vi "Customizing the Menubar.vi"() -> ()   [LabVIEW 2014]
doc: "本VI演示如何通过编程添加和删除VI运行时菜单栏中的项。"
uses:
  <vilib>/Utility/miscctls.llb/LVMenuShortCut.ctl
panel:
  in  "删除首选项":bool
  in  "删除新建":bool
  out "已选菜单项标识符":string
  in  "停止":bool
  # "概述：演示使用菜单函数控制VI运行时菜单栏的内容。\n操作步骤：\n1. 运行VI。自定义“文件”和“编辑”菜单将出现在菜单栏中。\n2. 选择多个不同菜单项。选择将显示在已选菜单项标识符显示控件中。\n3. 单击两个删除按钮。注意“文件 > 新建”和“文件 > 首选项”菜单项已移除。\n4. 单击停止可停止VI。"
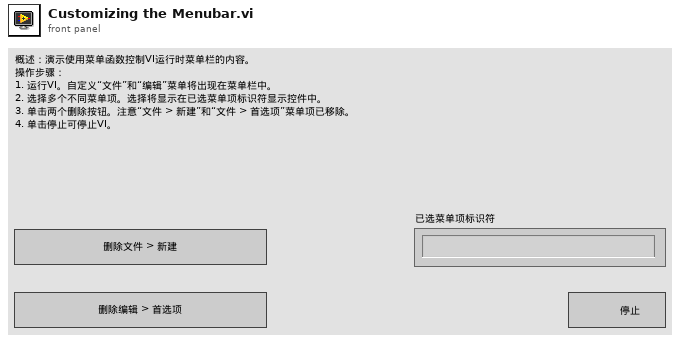
[diagram p1: front panel]
types:
  T1 = enum8{"Enabled", "Disabled", "Disabled and Grayed Out"}
  T2 = typedef "LVMenuShortCut.ctl" = cluster{"Include Shift Key?":bool, "Include Ctrl Key?":bool, "Shortcut Key":string}
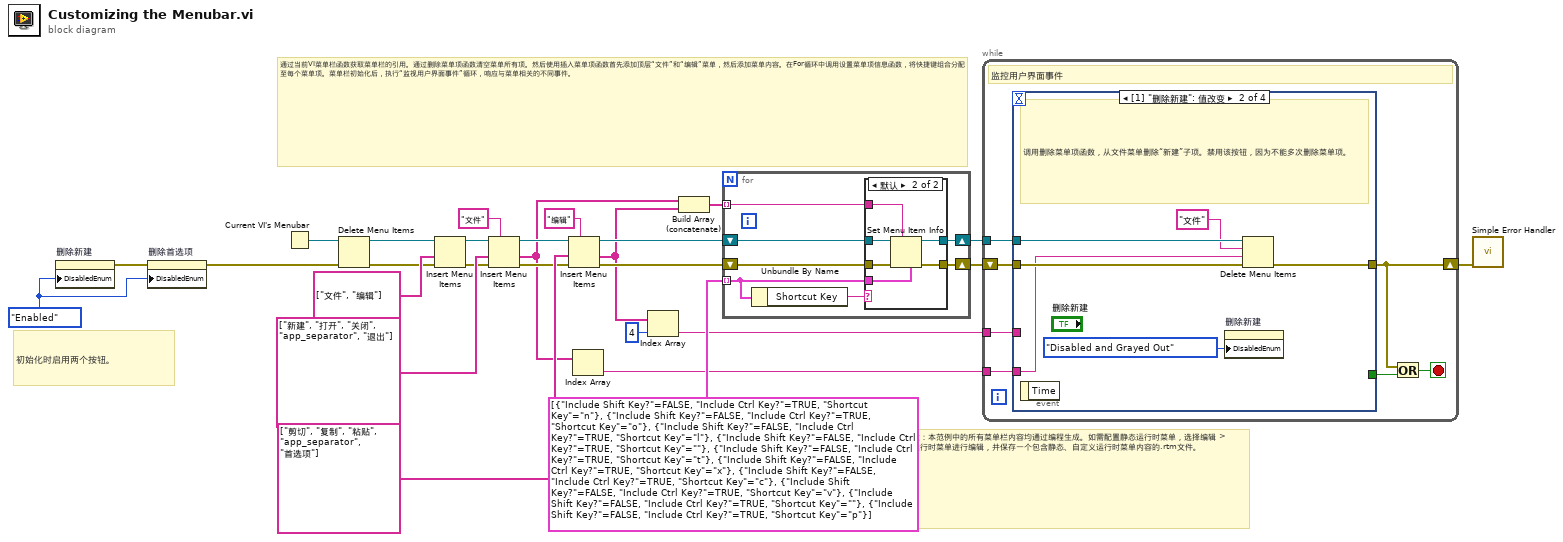
[diagram p0: block diagram]
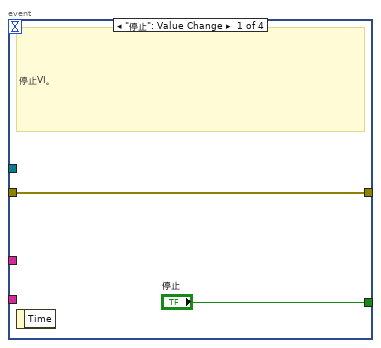
[diagram p2: hidden frame]
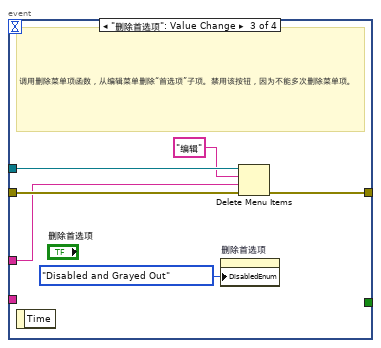
[diagram p3: hidden frame]
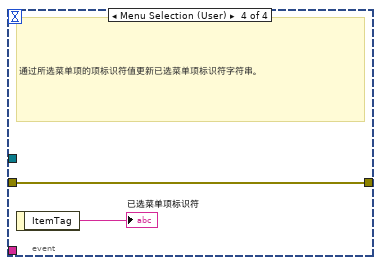
[diagram p4: hidden frame]
diagram:
  w1 = T1."Enabled" ("Disabled")
  # "注：本范例中的所有菜单栏内容均通过编程生成。如需配置静态运行时菜单，选择编辑 > 运行时菜单进行编辑，并保存一个包含静态、自定义运行时菜单内容的.rtm文件。"
  # "初始化时启用两个按钮。"
  # "通过当前VI菜单栏函数获取菜单栏的引用。通过删除菜单项函数清空菜单所有项。然后使用插入菜单项函数首先添加顶层“文件”和“编辑”菜单，然后添加菜单内容。在For循环中调用设置菜单项信息函数，将快捷键组合分配至每个菜单项。菜单栏初始化后，执行“监视用户界面事件”循环，响应与菜单相关的不同事件。"
  n1 = property on="删除新建" class="Bool"("DisabledEnum"=w1) -> (error out=w3:errorcluster)  [unwired: 2 in, 1 out]
  n2 = property on="删除首选项" class="Bool"(error in=w3, "DisabledEnum"=w1) -> (error out=w2:errorcluster)  [unwired: 1 in, 1 out]
  n3 = Current VI's Menubar() -> (w17:refnum<k9>)
  n4 = Delete Menu Items(6:w2, 9:w17) -> (0:w12:errorcluster, 3:w18:refnum<k9>)  [unwired: 2 in]
  n5 = Insert Menu Items(6:w12, 7:string[] ["文件", "编辑"] ("L10n_item tags 1"), 9:w18) -> (0:w16:errorcluster, 3:w27:refnum<k9>)  [unwired: 3 in, 1 out]
  n6 = Insert Menu Items(5:"文件" ("L10n_menu tag"), 6:w16, 7:string[] ["新建", "打开", "关闭", "app_separator", "退出"] ("L10n_item tags 2"), 9:w27) -> (0:w15:errorcluster, 1:w4:string[], 3:w26:refnum<k9>)  [unwired: 2 in]
  n7 = Insert Menu Items(5:"编辑" ("L10n_menu tag"), 6:w15, 7:string[] ["剪切", "复制", "粘贴", "app_separator", "首选项"] ("L10n_item tags 3"), 9:w26) -> (0:w14:errorcluster, 1:w7:string[], 3:w25:refnum<k9>)  [unwired: 2 in]
  n8 = Index Array(array=w4) -> (element=w8:string)  [unwired: 1 in]
  n9 = Index Array(array=w7, index=4) -> (element=w6:string)
  n10 = Build Array (concatenate)(w4, w7) -> (w21:string[])
  n11 = for {
    tunnel: w21 -> [w33] mode=indexing
    tunnel: T2[] [{"Include Shift Key?"=FALSE, "Include Ctrl Key?"=TRUE, "Shortcut Key"="n"}, {"Include Shift Key?"=FALSE, "Include Ctrl Key?"=TRUE, "Shortcut Key"="o"}, {"Include Shift Key?"=FALSE, "Include Ctrl Key?"=TRUE, "Shortcut Key"="l"}, {"Include Shift Key?"=FALSE, "Include Ctrl Key?"=TRUE, "Shortcut Key"=""}, {"Include Shift Key?"=FALSE, "Include Ctrl Key?"=TRUE, "Shortcut Key"="t"}, {"Include Shift Key?"=FALSE, "Include Ctrl Key?"=TRUE, "Shortcut Key"="x"}, {"Include Shift Key?"=FALSE, "Include Ctrl Key?"=TRUE, "Shortcut Key"="c"}, {"Include Shift Key?"=FALSE, "Include Ctrl Key?"=TRUE, "Shortcut Key"="v"}, {"Include Shift Key?"=FALSE, "Include Ctrl Key?"=TRUE, "Shortcut Key"=""}, {"Include Shift Key?"=FALSE, "Include Ctrl Key?"=TRUE, "Shortcut Key"="p"}] -> [w29] mode=indexing
    shift-right: [w31] -> w13
    shift-left: w14 -> [w32]
    shift-right: [w30] -> w9
    shift-left: w25 -> [w34]
    n12 = Unbundle By Name(w29) -> ("Shortcut Key"=w28:string)
    n13 = case shown="默认" w28 {
      tunnel: w34 -> [w36 w42]
      tunnel: w33 -> [_ w41]
      tunnel: w32 -> [w35 w40]
      tunnel: [w35 w39] -> w31
      tunnel: [w36 w38] -> w30
      tunnel: w29 -> [_ w37]
      frame "" {
      }
      frame Default {
        n14 = Set Menu Item Info(4:w37, 7:w41, 8:w40, 11:w42) -> (0:w39:errorcluster, 3:w38:refnum<k9>)  [unwired: 3 in]
      }
    }
  }
  n15 = while {
    shift-right: [w46] -> w10
    shift-left: w13 -> [w49]
    tunnel: w9 -> [w45]
    tunnel: w8 -> [w44]
    tunnel: w6 -> [w43]
    stop <- w47 stop-if-true
    # "监控用户界面事件"
    n16 = event shown="[1] \"删除新建\": 值改变" {
      selector: _ -> [_ _ _ _]
      dyn-events: _ -> [_ _ _ _]
      timeout: _ -> [_ _ _ _]
      tunnel: w49 -> [w51 w56 w62 w64]
      tunnel: [w51 w57 w63 w64] -> w46
      tunnel: ["停止" _ _ _] -> w48
      tunnel: w45 -> [_ w55 w61 _]
      tunnel: w44 -> [_ w53 _ _]
      tunnel: w43 -> [_ _ w59 _]
      event "停止": Value Change {
        # "停止VI。"
        n17 = event-data() -> ()  [unwired: 1 in, 1 out]
      }
      event "删除新建": Value Change {
        # "调用删除菜单项函数，从文件菜单删除“新建”子项。禁用该按钮，因为不能多次删除菜单项。"
        n18 = event-data() -> ()  [unwired: 1 in, 1 out]
        n19 = property on="删除新建" class="Bool"("DisabledEnum"=T1."Disabled and Grayed Out" ("Disabled")) -> ()  [unwired: 2 in, 2 out]
        n20 = Delete Menu Items(6:w56, 7:w53, 8:"文件" ("L10n_menu tag"), 9:w55) -> (0:w57:errorcluster)  [unwired: 1 out]
      }
      event "删除首选项": Value Change {
        # "调用删除菜单项函数，从编辑菜单删除“首选项”子项。禁用该按钮，因为不能多次删除菜单项。"
        n21 = event-data() -> ()  [unwired: 1 in, 1 out]
        n22 = property on="删除首选项" class="Bool"("DisabledEnum"=T1."Disabled and Grayed Out" ("Disabled")) -> ()  [unwired: 2 in, 2 out]
        n23 = Delete Menu Items(6:w62, 7:w59, 8:"编辑" ("L10n_menu tag"), 9:w61) -> (0:w63:errorcluster)  [unwired: 1 out]
      }
      event Menu Selection (User) {
        # "通过所选菜单项的项标识符值更新已选菜单项标识符字符串。"
        n24 = event-data() -> ("ItemTag"=→"已选菜单项标识符":string)  [unwired: 1 in]
      }
    }
    n25 = Or(x=w46, y=w48) -> (x .or. y?=w47:bool)
  }
  n26 = call <vilib>:"Simple Error Handler.vi"("error in (no error)"=w10) -> ()  [unwired: 4 in, 5 out]
